vi "LF_Tester_RCstage_dbTester_Cmb.vi"() -> ()   [LabVIEW 2017]
uses:
  <vilib>/userdefined/High Color/IMAQdx.ctl
panel:
  in  "Tab Control":enum32{"Front Stage", "Back Stage"}(tab)=enum."Back Stage"
  in  "Spectrometer Data Front":path=path "C:/Life_Tester_Proj/Life_Tester_Proj/labVIEW_proj/TestData/20190627_dbRCstage/Front/spectrum.txt"
  in  "Emitter Image Data Front":path=path "C:/Life_Tester_Proj/Life_Tester_Proj/labVIEW_proj/TestData/20190627_dbRCstage/Front/emitter.txt"
  in  "Select Camera Front":T1="lfCam_Front"
  in  "Power Meter Data Front":path=path "C:/Life_Tester_Proj/Life_Tester_Proj/labVIEW_proj/TestData/20190627_dbRCstage/Front/power.txt"
  in  "Current(A) Input Front":dbl=291.8 format="%#_13g"
  in  "Illasco_SN Front":string[](array[string])=["LF_15", "LF_14", "LF_13", "LF_12", "LF_11", "LF_10", "LF_9", "LF_8", "LF_7", "LF_6", "LF_5", "LF_4", "LF_3", "LF_2", "LF_1"]
  in  "Power Meter Front":enum16{"Front", "Back"}(ring)
  in  "Spectrometer Front":enum16{"Front", "Back"}(ring)
  in  "Stage Ref. In Front":refnum<visa-resource-name>="Lf_Tester_Stage_Front"
  in  "Spectrometer Data Back":path=path "C:/Life_Tester_Proj/Life_Tester_Proj/labVIEW_proj/TestData/20190627_dbRCstage/Back/spectrum.txt"
  in  "Emitter Image Back":path=path "C:/Life_Tester_Proj/Life_Tester_Proj/labVIEW_proj/TestData/20190627_dbRCstage/Back/emitter.txt"
  in  "Select Camera Back":T1="lfCam_Back"
  in  "Power Meter Data Back":path=path "C:/Life_Tester_Proj/Life_Tester_Proj/labVIEW_proj/TestData/20190627_dbRCstage/Back/power.txt"
  in  "Current(A) Input Back":dbl=291.8 format="%#_13g"
  in  "Illasco_SN Back":string[](array[string])=["LF_15", "LF_14", "LF_13", "LF_12", "LF_11", "LF_10", "LF_9", "LF_8", "LF_7", "LF_6", "LF_5", "LF_4", "LF_3", "LF_2", "LF_1"]
  in  "Power Meter Back":enum16{"Front", "Back"}(ring)=enum."Back"
  in  "Spectrometer Back":enum16{"Front", "Back"}(ring)=enum."Back"
  in  "Stage Ref. In Back":refnum<visa-resource-name>="Lf_Tester_Stage_Back"
  # "Initialization Front"
  # "Initialization Back"
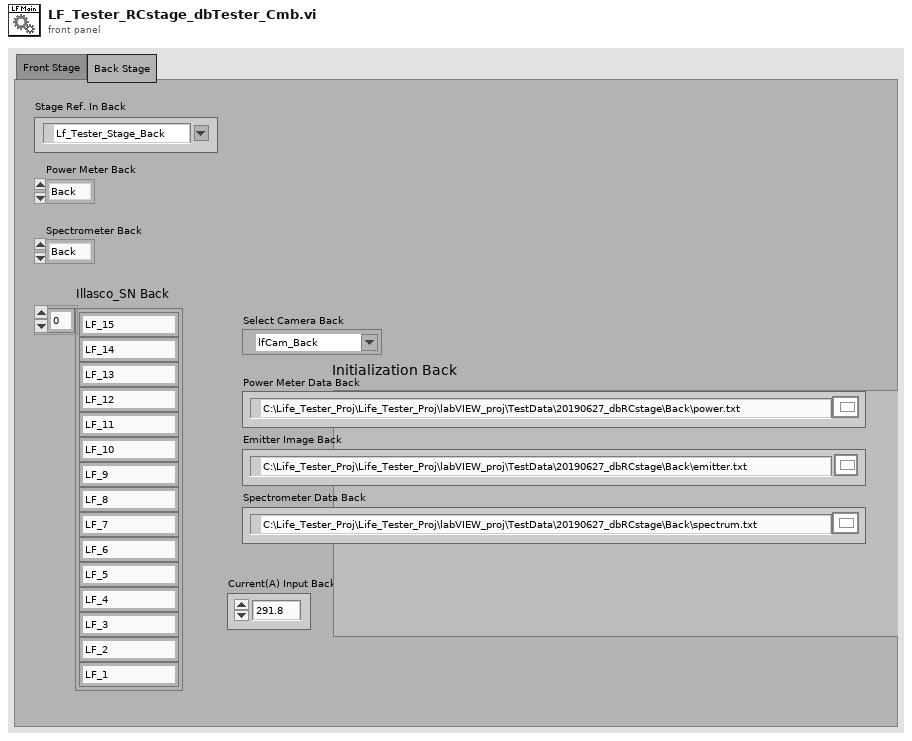
[diagram p1: front panel]
types:
  T1 = typedef "IMAQdx.ctl" = refnum<k21>
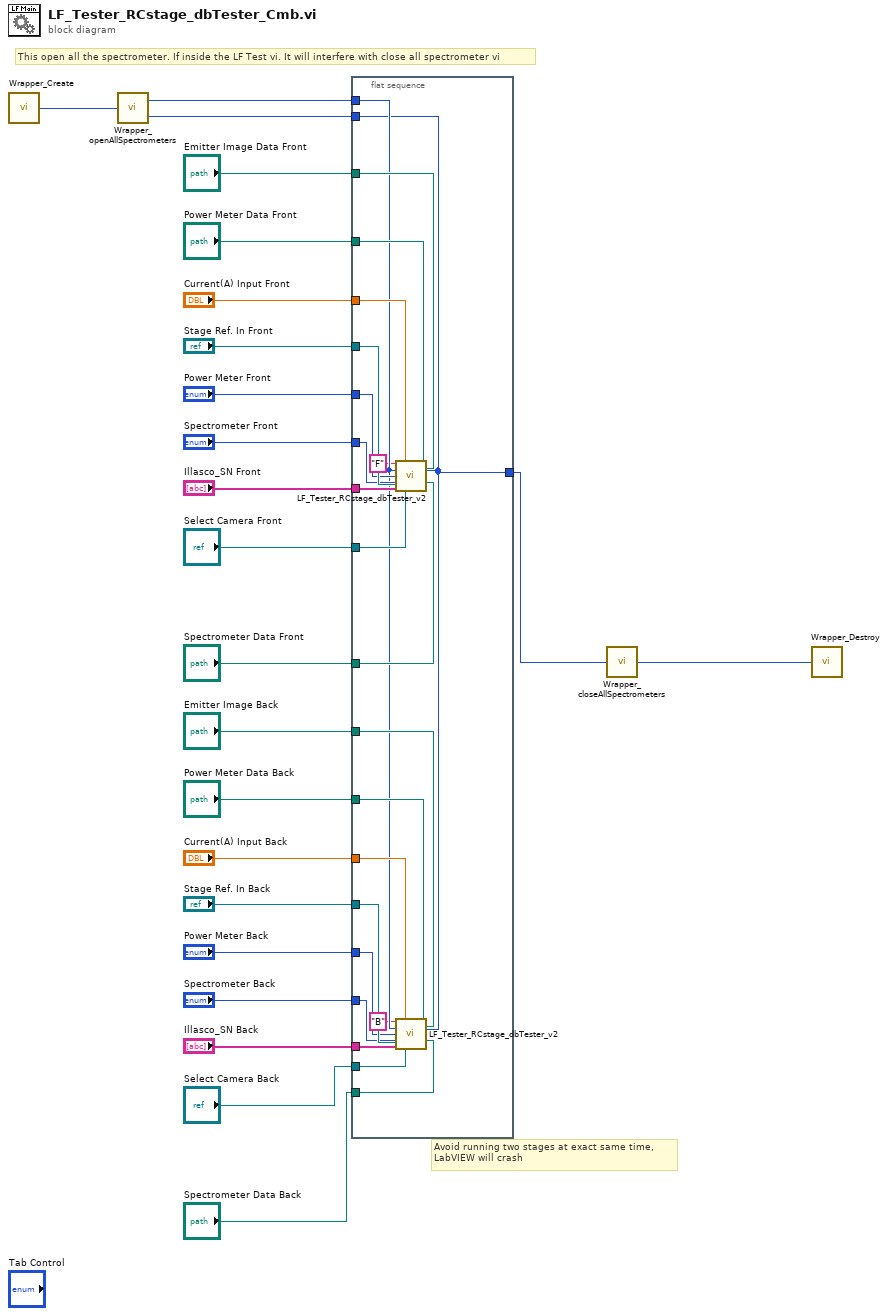
[diagram p0: block diagram]
diagram:
  # "This open all the spectrometer. If inside the LF Test vi. It will interfere with close all spectrometer vi"
  # "Avoid running two stages at exact same time, \nLabVIEW will crash"
  n1 = call "Wrapper_Create.vi"() -> ("Wrapper"=w5:u32)
  n2 = call "Wrapper_openAllSpectrometers.vi"("Wrapper In"=w5) -> ("Number of Spectrometers"=w4:i32, "Wrapper Out"=w3:u32)
  n3 = flat-sequence {
    tunnel: "Stage Ref. In Front" -> [w45]
    tunnel: "Power Meter Front" -> [w44]
    tunnel: "Spectrometer Front" -> [w43]
    tunnel: "Illasco_SN Front" -> [w42]
    tunnel: "Select Camera Front" -> [w41]
    tunnel: "Power Meter Data Front" -> [w40]
    tunnel: "Emitter Image Data Front" -> [w39]
    tunnel: "Spectrometer Data Front" -> [w38]
    tunnel: "Current(A) Input Front" -> [w37]
    tunnel: "Stage Ref. In Back" -> [w36]
    tunnel: "Power Meter Back" -> [w35]
    tunnel: "Spectrometer Back" -> [w34]
    tunnel: "Illasco_SN Back" -> [w33]
    tunnel: "Select Camera Back" -> [w32]
    tunnel: "Power Meter Data Back" -> [w31]
    tunnel: "Emitter Image Back" -> [w30]
    tunnel: "Spectrometer Data Back" -> [w29]
    tunnel: "Current(A) Input Back" -> [w28]
    tunnel: w4 -> [w27]
    tunnel: w3 -> [w26]
    tunnel: [w26] -> w1
    frame #0 {
      n4 = call "LF_Tester_RCstage_dbTester_v2.vi"("string"="F", "Current(A) Input"=w37, "Emitter Image Data"=w39, "Power Meter Data File"=w40, "Number of Spectrometers"=w27, "Wrapper In"=w26, "Power Meter"=w44, "Spectrometer"=w43, "Spectrometer Data File"=w38, "Illasco_SN"=w42, "Select Camera"=w41, "Stage Ref. In"=w45) -> ()  [unwired: 4 in]
      n5 = call "LF_Tester_RCstage_dbTester_v2.vi"("string"="B", "Current(A) Input"=w28, "Emitter Image Data"=w30, "Power Meter Data File"=w31, "Number of Spectrometers"=w27, "Wrapper In"=w26, "Power Meter"=w35, "Spectrometer"=w34, "Spectrometer Data File"=w29, "Illasco_SN"=w33, "Select Camera"=w32, "Stage Ref. In"=w36) -> ()  [unwired: 4 in]
    }
  }
  n6 = call "Wrapper_closeAllSpectrometers.vi"("Wrapper In"=w1) -> ("Wrapper Out"=w2:u32)
  n7 = call "Wrapper_Destroy.vi"("Wrapper"=w2) -> ()
